vi "FreqPwrMeasureConfig.vi"(7 "Freq/Pwr":T1, 8 "error in (no error)":errorcluster, 11 "FreqMeasureConfig":T3={"TriggerSource"=enum."RIO0", "ReferenceLevel"=0.0, "Freq"=0.0, "PhyPort"=enum."Port5"}) -> (0 "error out":errorcluster, 3 "FreqMeasureConfig":string[](array[string]))   [LabVIEW 2015]
uses:
  PhyPort.ctl
  PwrFreq.ctl
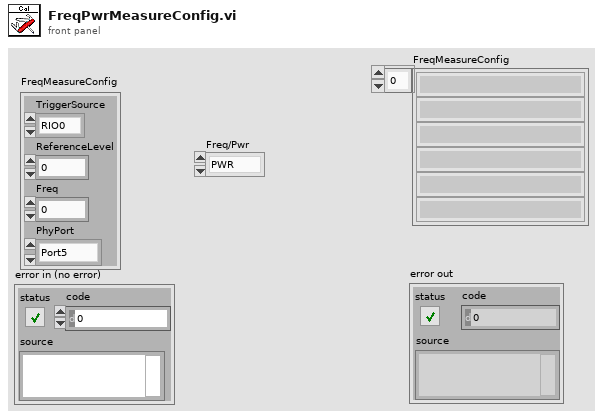
[diagram p1: front panel]
types:
  T1 = typedef "PwrFreq.ctl" = enum16{"PWR", "FREQ"}
  T2 = typedef "PhyPort.ctl" = enum16{"Port0", "Port1", "Port2", "Port3", "Port4", "Port5", "Port6", "Port7"}
  T3 = cluster{"TriggerSource":enum16{"RIO0", "RIO1"}, "ReferenceLevel":dbl, "Freq":dbl, "PhyPort":T2}
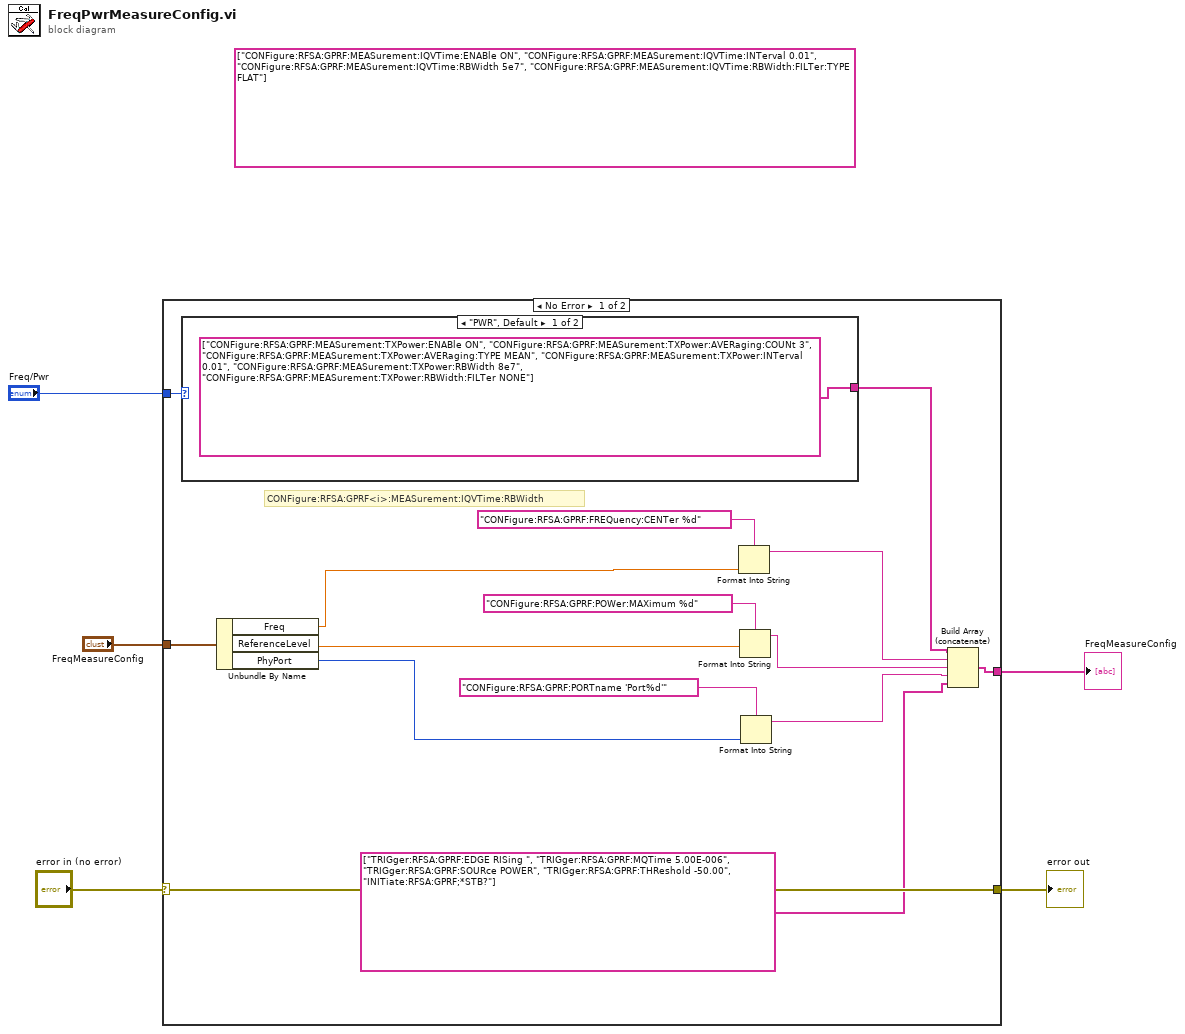
[diagram p0: block diagram]
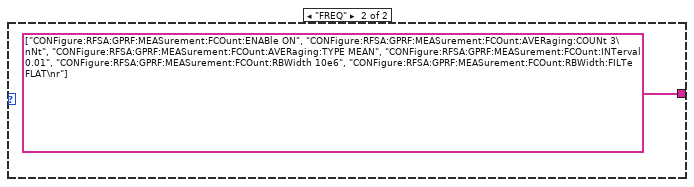
[diagram p2: hidden frame]
diagram:
  (unwired) string[] ["CONFigure:RFSA:GPRF:MEASurement:IQVTime:ENABle ON", "CONFigure:RFSA:GPRF:MEASurement:IQVTime:INTerval 0.01", "CONFigure:RFSA:GPRF:MEASurement:IQVTime:RBWidth 5e7", "CONFigure:RFSA:GPRF:MEASurement:IQVTime:RBWidth:FILTer:TYPE FLAT"]
  n1 = case shown="No Error" "error in (no error)" {
    selector: "error in (no error)" -> [w13 w23]
    tunnel: [w16 _] -> w5
    tunnel: "FreqMeasureConfig" -> [w15 _]
    tunnel: [w13 w23] -> w2
    tunnel: "Freq/Pwr" -> [w8 _]
    frame No Error {
      # "CONFigure:RFSA:GPRF<i>:MEASurement:IQVTime:RBWidth"
      n2 = case shown="\"PWR\", Default" w8 {
        tunnel: [string[] ["CONFigure:RFSA:GPRF:MEASurement:TXPower:ENABle ON", "CONFigure:RFSA:GPRF:MEASurement:TXPower:AVERaging:COUNt 3", "CONFigure:RFSA:GPRF:MEASurement:TXPower:AVERaging:TYPE MEAN", "CONFigure:RFSA:GPRF:MEASurement:TXPower:INTerval 0.01", "CONFigure:RFSA:GPRF:MEASurement:TXPower:RBWidth 8e7", "CONFigure:RFSA:GPRF:MEASurement:TXPower:RBWidth:FILTer NONE"] string[] ["CONFigure:RFSA:GPRF:MEASurement:FCOunt:ENABle ON", "CONFigure:RFSA:GPRF:MEASurement:FCOunt:AVERaging:COUNt 3\nNt", "CONFigure:RFSA:GPRF:MEASurement:FCOunt:AVERaging:TYPE MEAN", "CONFigure:RFSA:GPRF:MEASurement:FCOunt:INTerval 0.01", "CONFigure:RFSA:GPRF:MEASurement:FCOunt:RBWidth 10e6", "CONFigure:RFSA:GPRF:MEASurement:FCOunt:RBWidth:FILTe FLAT\nr"]] -> w10
        frame "PWR", Default {
        }
        frame "FREQ" {
        }
      }
      n3 = Unbundle By Name(w15) -> ("Freq"=w11:dbl, "ReferenceLevel"=w14:dbl, "PhyPort"=w6:T2)
      n4 = Format Into String(format string="CONFigure:RFSA:GPRF:FREQuency:CENTer %d", w11) -> (resulting string=w9:string)  [unwired: 2 in, 1 out]
      n5 = Format Into String(format string="CONFigure:RFSA:GPRF:POWer:MAXimum %d", w14) -> (resulting string=w18:string)  [unwired: 2 in, 1 out]
      n6 = Format Into String(format string="CONFigure:RFSA:GPRF:PORTname 'Port%d'", w6) -> (resulting string=w17:string)  [unwired: 2 in, 1 out]
      n7 = Build Array (concatenate)(w10, w9, w18, w17, string[] ["TRIGger:RFSA:GPRF:EDGE RISing ", "TRIGger:RFSA:GPRF:MQTime 5.00E-006", "TRIGger:RFSA:GPRF:SOURce POWER", "TRIGger:RFSA:GPRF:THReshold -50.00", "INITiate:RFSA:GPRF;*STB?"]) -> (w16:string[])
    }
    frame Error {
    }
  }
  "FreqMeasureConfig" <- w5
  "error out" <- w2
